vi "Update Build Spec Destination Name with Version.vi"(8 "error in (no error)":errorcluster, 10 "Search Pattern":string, 11 "LabVIEW Build Script in":refnum<class "LabVIEW Build Script.lvclass">) -> (0 "error out":errorcluster, 3 "LabVIEW Build Script out":refnum<class "LabVIEW Build Script.lvclass">)   [LabVIEW 2021, in "LabVIEW Build Script.lvclass"]
uses:
  LabVIEW Build Script.lvclass
  LabVIEW Build Script.lvclass/LabVIEW Build Script.ctl
  <vilib>/CIF Foundation/CIF Utilities/Errors/Errors_CIF_U.lvlib
  Build Script Common/Typedef/Build Script Errors.ctl
  Build Script Common/Build Script Common.lvlib
  <vilib>/CIF Foundation/CIF LabVIEW Scripting/LV Scripting/LV Scripting Utilities.lvlib
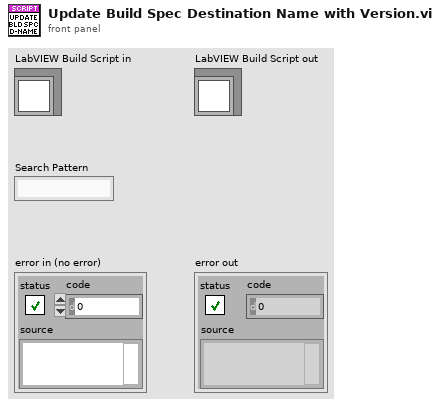
[diagram p1: front panel]
types:
  T1 = typedef "Build Script Common.lvlib/Build Script Errors.ctl" = enum16{"Item not found"}
  T2 = typedef "LV Scripting Utilities.lvlib/BuildSpec Map.ctl" = map{string, refnum<vi>}
  T3 = typedef "LV Scripting Utilities.lvlib/Library Map.ctl" = map{string, refnum<vi>}
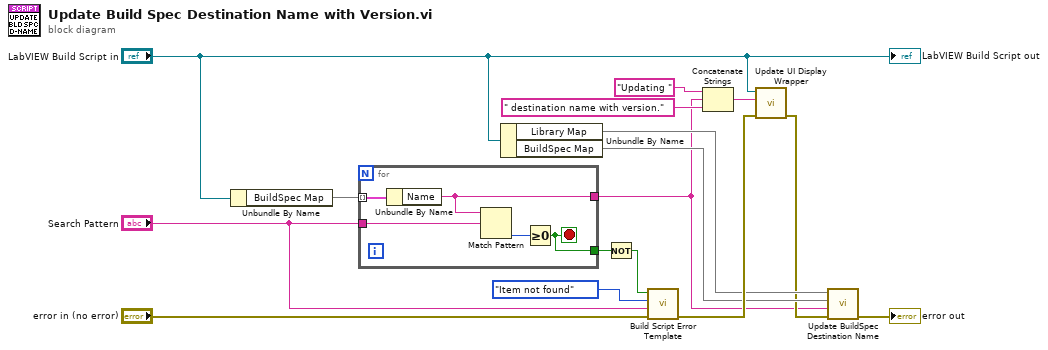
[diagram p0: block diagram]
diagram:
  n1 = Unbundle By Name("LabVIEW Build Script in") -> ("BuildSpec Map"=w13:T2)
  n2 = for {
    tunnel: w13 -> [w21] mode=indexing
    tunnel: "Search Pattern" -> [w20]
    tunnel: [w18] -> w2
    tunnel: [w17] -> w11
    stop <- w17 stop-if-true
    n3 = Unbundle By Name(w21) -> ("Name"=w18:string)
    n4 = Match Pattern(string=w18, regular expression=w20) -> (offset past match=w19:i32)  [unwired: 1 in, 3 out]
    n5 = Greater Or Equal To 0?(x=w19) -> (x >= 0?=w17:bool)
  }
  n6 = Unbundle By Name("LabVIEW Build Script in") -> ("Library Map"=w5:T3, "BuildSpec Map"=w4:T2)
  n7 = Not(x=w11) -> (.not. x?=w10:bool)
  n8 = call "Build Script Error Template.vi"("error in (no error)"="error in (no error)", "String to Append"="Search Pattern", "Error"=Build_Script_Errors."Item not found", "Insert Error"=w10) -> ("error out"=w6:errorcluster)  [unwired: 7 in]
  n9 = Concatenate Strings("Updating " ("Update for Display"), w2, " destination name with version." ("string")) -> (w15:string)
  n10 = call "Update UI Display Wrapper.vi"("error in (no error)"=w6, "Update for Display"=w15, "LabVIEW Build Script in"="LabVIEW Build Script in") -> ("error out"=w3:errorcluster)  [unwired: 8 in]
  n11 = call <vilib>:"Update BuildSpec Destination Name.vi"("error in (no error)"=w3, "BuildSpec Name"=w2, "BuildSpec Map"=w4, "Library Map"=w5) -> ("error out"=→"error out":errorcluster)  [unwired: 7 in]
  "LabVIEW Build Script out" <- "LabVIEW Build Script in"
